vi "Cache_Path Global.vi"() -> ()   [LabVIEW 2019, in "ClassLoader.lvlib"]
uses:
  ClassLoader.lvlib
panel:
  in  "Path map":map{string, path}(c390)
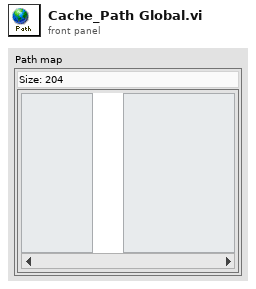
[diagram p1: front panel]
diagram:
